vi "Arrange Displays DEMO.vi"() -> ()   [LabVIEW 2016]
uses:
  <vilib>/Utility/miscctls.llb/LVPointTypeDef.ctl
panel:
  in  "stop":bool
  in  "Number of Displays":u8
  in  "Aspect Ratio (Width/Height)":dbl
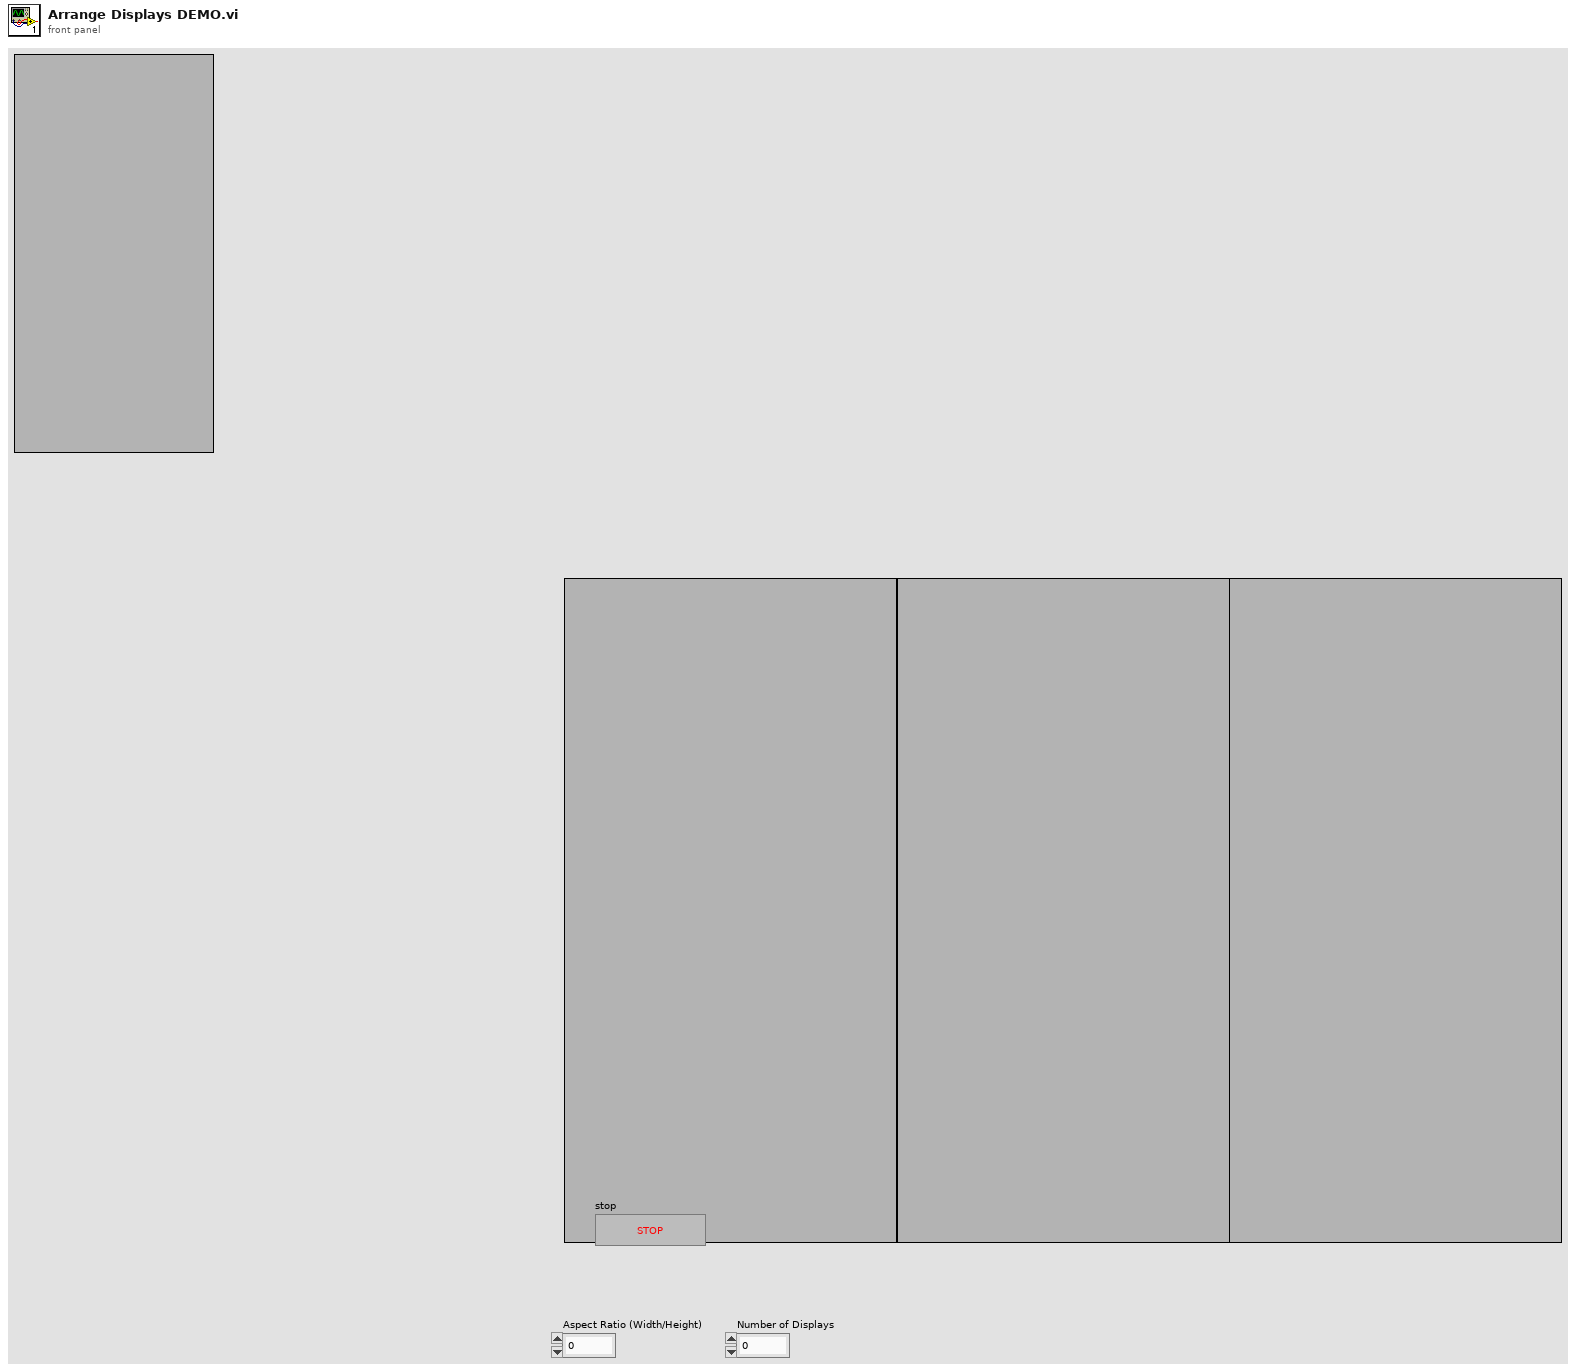
[diagram p1: front panel]
types:
  T1 = enum16{"Always On", "Always Off", "Off While Running"}
  T2 = typedef "LVPointTypeDef.ctl" = cluster{"Horizontal":i16, "Vertical":i16}
  T3 = typedef "LVRectTypeDef.ctl" = cluster{"Left":i16, "Top":i16, "Right":i16, "Bottom":i16}
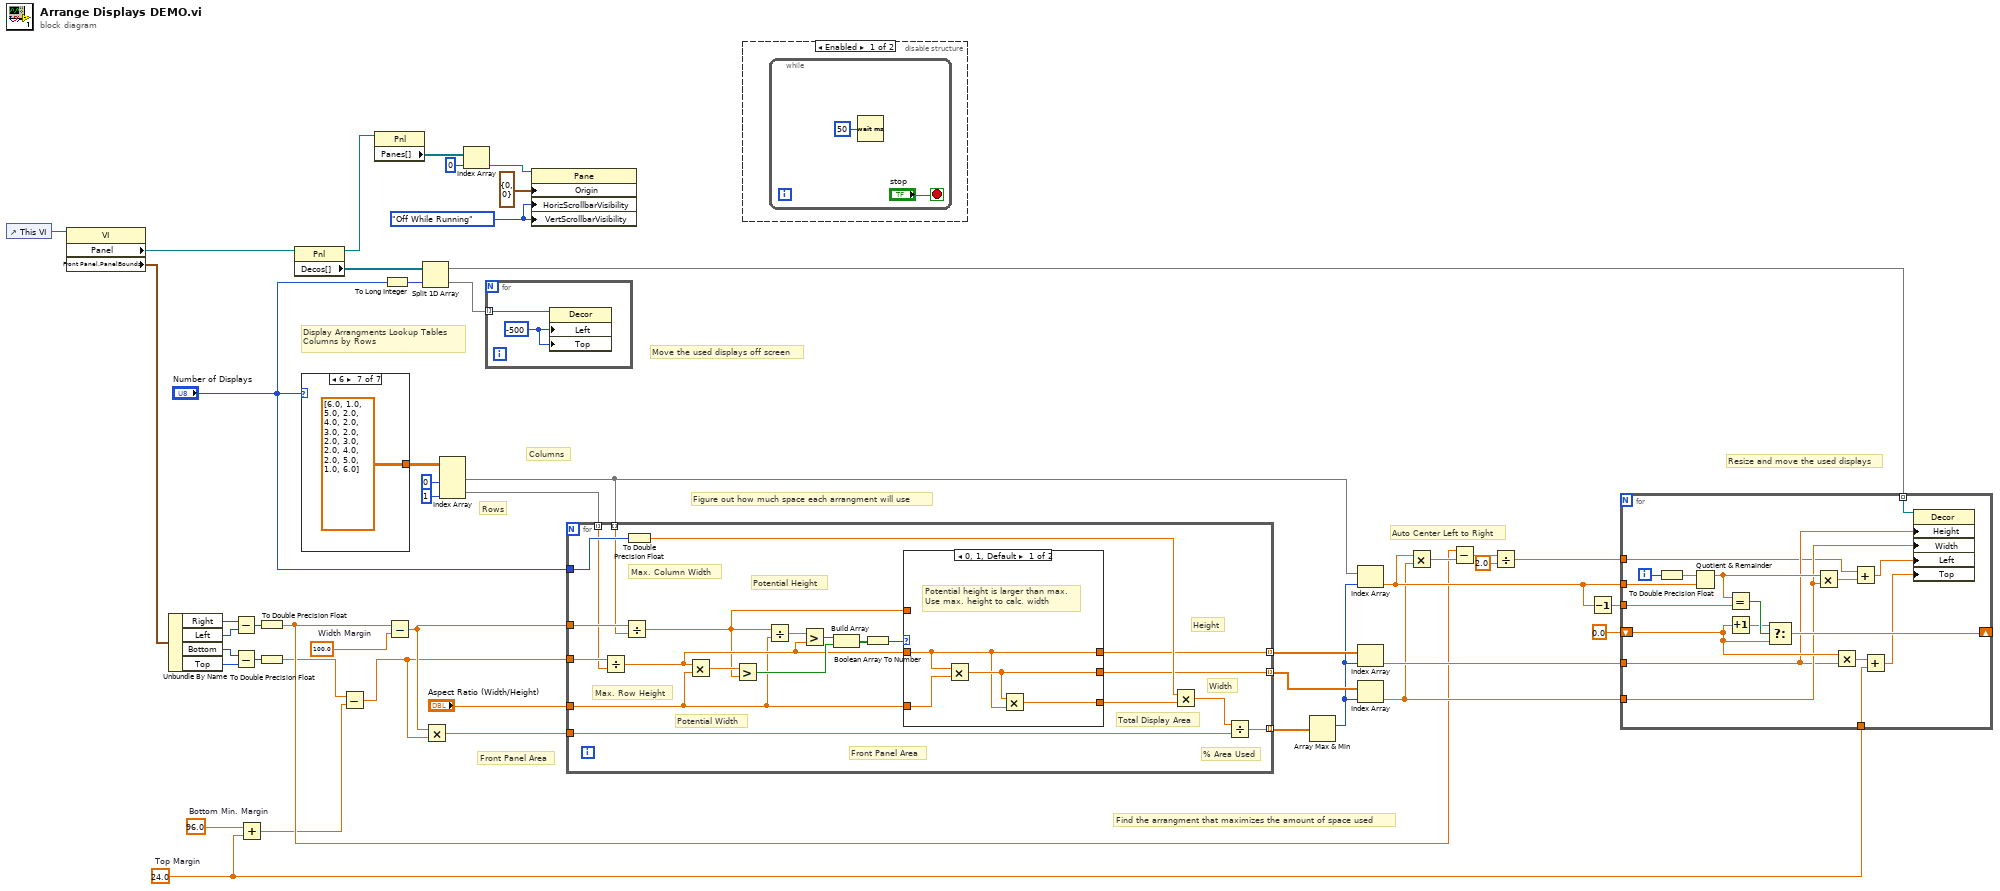
[diagram p0: block diagram]
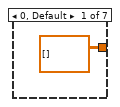
[diagram p3: hidden frame]
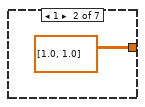
[diagram p4: hidden frame]
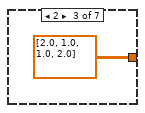
[diagram p5: hidden frame]
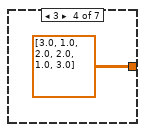
[diagram p6: hidden frame]
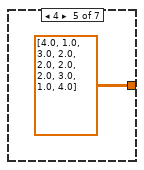
[diagram p7: hidden frame]
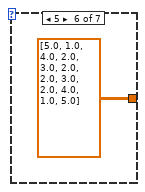
[diagram p8: hidden frame]
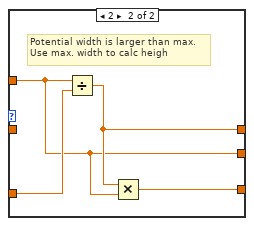
[diagram p9: hidden frame]
diagram:
  w1 = 96.0  # Bottom Min. Margin
  w5 = 24.0  # Top Margin
  w14 = 100.0  # Width Margin
  w42 = T1."Off While Running" ("Vertical Scrollbar Visibility")
  # "Auto Center Left to Right"
  # "Resize and move the used displays"
  # "Find the arrangment that maximizes the amount of space used"
  # "Figure out how much space each arrangment will use"
  # "Move the used displays off screen"
  # "Front Panel Area"
  # "Rows"
  # "Columns"
  # "Display Arrangments Lookup Tables\nColumns by Rows"
  n1 = control-ref of="This VI"() -> (w48:refnum<vi>)
  n2 = property class="VI"(reference=w48) -> ("Panel"=w47:refnum<vi>, "Front Panel.PanelBounds"=w40:T3)  [unwired: 1 in, 2 out]
  n3 = Unbundle By Name(w40) -> ("Right"=w39:i16, "Left"=w38:i16, "Bottom"=w37:i16, "Top"=w36:i16)
  n4 = Subtract(x=w39, y=w38) -> (x-y=w34:i16)
  n5 = Subtract(x=w37, y=w36) -> (x-y=w33:i16)
  n6 = Add(x=w1, y=w5) -> (x+y=w4:dbl)
  n7 = To Double Precision Float(number=w34) -> (double precision float=w6:dbl)
  n8 = To Double Precision Float(number=w33) -> (double precision float=w3:dbl)
  n9 = property class="Pnl"(reference=w47) -> (reference out=w41:refnum<vi>, "Decos[]"=w19:refnum<vi>[])  [unwired: 1 in, 1 out]
  n10 = case shown="6" "Number of Displays" {
    tunnel: [dbl[][] [] dbl[][] [[1.0, 1.0]] dbl[][] [[2.0, 1.0], [1.0, 2.0]] dbl[][] [[3.0, 1.0], [2.0, 2.0], [1.0, 3.0]] dbl[][] [[4.0, 1.0], [3.0, 2.0], [2.0, 2.0], [2.0, 3.0], [1.0, 4.0]] dbl[][] [[5.0, 1.0], [4.0, 2.0], [3.0, 2.0], [2.0, 3.0], [2.0, 4.0], [1.0, 5.0]] dbl[][] [[6.0, 1.0], [5.0, 2.0], [4.0, 2.0], [3.0, 2.0], [2.0, 3.0], [2.0, 4.0], [2.0, 5.0], [1.0, 6.0]]] -> w31
    frame 0, Default {
    }
    frame 1 {
    }
    frame 2 {
    }
    frame 3 {
    }
    frame 4 {
    }
    frame 5 {
    }
    frame 6 {
    }
  }
  n11 = Subtract(x=w3, y=w4) -> (x-y=w2:dbl)
  n12 = property class="Pnl"(reference=w41) -> ("Panes[]"=w46:refnum<vi>[])  [unwired: 1 in, 2 out]
  n13 = To Long Integer(number="Number of Displays") -> (32bit integer=w17:i32)
  n14 = Subtract(x=w6, y=w14) -> (x-y=w13:dbl)
  n15 = Split 1D Array(array=w19, index=w17) -> (first subarray=w18:refnum<vi>[], second subarray=w16:refnum<vi>[])
  n16 = Multiply(x=w13, y=w2) -> (x*y=w32:dbl)
  n17 = Index Array(array=w31, index (col) #1=0 ("disabled index (col)"), index (col) #2=1 ("index (col)")) -> (element #1=w24:dbl[], element #2=w23:dbl[])  [unwired: 2 in]
  n18 = Index Array(array=w46, index=0) -> (element=w44:refnum<vi>)
  n19 = for {
    tunnel: w16 -> [w57] mode=indexing
    w56 = -500 ("Position:Left")
    n20 = property class="Decor"(reference=w57, "Left"=w56, "Top"=w56) -> ()  [unwired: 1 in, 2 out]
  }
  n21 = property class="Pane"(reference=w44, "Origin"=T2 {"Horizontal"=0, "Vertical"=0}, "HorizScrollbarVisibility"=w42, "VertScrollbarVisibility"=w42) -> ()  [unwired: 1 in, 2 out]
  n22 = for {
    tunnel: "Aspect Ratio (Width/Height)" -> [w69]
    tunnel: w13 -> [w78]
    tunnel: w2 -> [w77]
    tunnel: w32 -> [w63]
    tunnel: [w66] -> w27 mode=indexing
    tunnel: [w65] -> w26 mode=indexing
    tunnel: [w62] -> w28 mode=indexing
    tunnel: w24 -> [w59] mode=indexing
    tunnel: w23 -> [w58] mode=indexing
    tunnel: "Number of Displays" -> [w60]
    # "% Area Used"
    # "Front Panel Area"
    # "Total Display Area"
    # "Width"
    # "Height"
    # "Potential Height"
    # "Potential Width"
    # "Max. Row Height"
    # "Max. Column Width"
    n23 = Divide(x=w77, y=w58) -> (x/y=w71:dbl)
    n24 = Divide(x=w78, y=w59) -> (x/y=w70:dbl)
    n25 = To Double Precision Float(number=w60) -> (double precision float=w67:dbl)
    n26 = Multiply(x=w71, y=w69) -> (x*y=w76:dbl)
    n27 = Greater?(x=w76, y=w70) -> (0:w73:bool)
    n28 = Divide(x=w70, y=w69) -> (x/y=w75:dbl)
    n29 = Greater?(x=w75, y=w71) -> (0:w74:bool)
    n30 = Build Array(w74, w73) -> (w72:bool[])
    n31 = Boolean Array To Number(Boolean array=w72) -> (number=w61:u32)
    n32 = case shown="0, 1, Default" w61 {
      tunnel: w71 -> [w80 _]
      tunnel: w70 -> [_ w84]
      tunnel: w69 -> [w82 w86]
      tunnel: [w80 w85] -> w66
      tunnel: [w81 w84] -> w65
      tunnel: [w79 w83] -> w68
      frame 0, 1, Default {
        # "Potential height is larger than max.\nUse max. height to calc. width"
        n33 = Multiply(x=w80, y=w82) -> (x*y=w81:dbl)
        n34 = Multiply(x=w81, y=w80) -> (x*y=w79:dbl)
      }
      frame 2 {
        # "Potential width is larger than max.\nUse max. width to calc heigh"
        n35 = Divide(x=w84, y=w86) -> (x/y=w85:dbl)
        n36 = Multiply(x=w85, y=w84) -> (x*y=w83:dbl)
      }
    }
    n37 = Multiply(x=w67, y=w68) -> (x*y=w64:dbl)
    n38 = Divide(x=w64, y=w63) -> (x/y=w62:dbl)
  }
  n39 = disable-structure shown="Enabled" {
    frame Enabled {
      n40 = while {
        stop <- "stop" stop-if-true
        n41 = Wait (ms)(milliseconds to wait=u32 50) -> ()  [unwired: 1 out]
      }
    }
    frame Disabled {
    }
  }
  n42 = Array Max & Min(array=w28) -> (max index (indices)=w22:i32)  [unwired: 3 out]
  n43 = Index Array(array=w24, index=w22) -> (element=w12:dbl)
  n44 = Index Array(array=w27, index=w22) -> (element=w25:dbl)
  n45 = Index Array(array=w26, index=w22) -> (element=w11:dbl)
  n46 = Multiply(x=w12, y=w11) -> (x*y=w10:dbl)
  n47 = Subtract(x=w6, y=w10) -> (x-y=w9:dbl)
  n48 = Divide(x=w9, y=2.0) -> (x/y=w7:dbl)
  n49 = Decrement(x=w12) -> (x-1=w21:dbl)
  n50 = for {
    tunnel: w25 -> [w95]
    tunnel: w11 -> [w96]
    tunnel: w12 -> [w106]
    tunnel: w18 -> [w97] mode=indexing
    tunnel: w21 -> [w103]
    shift-right: [w100] -> _
    shift-left: 0.0 -> [w99]
    tunnel: w7 -> [w93]
    tunnel: w5 -> [w90]
    i -> [w104]
    n51 = To Double Precision Float(number=w104) -> (double precision float=w105:dbl)
    n52 = Quotient & Remainder(x=w105, y=w106) -> (x-y*floor(x/y)=w98:dbl)  [unwired: 1 out]
    n53 = Equal?(x=w98, y=w103) -> (x = y?=w102:bool)
    n54 = Increment(x=w99) -> (x+1=w101:dbl)
    n55 = Select(t=w101, s=w102, f=w99) -> (s? t:f=w100:dbl)
    n56 = Multiply(x=w98, y=w96) -> (x*y=w94:dbl)
    n57 = Multiply(x=w99, y=w95) -> (x*y=w91:dbl)
    n58 = Add(x=w93, y=w94) -> (x+y=w92:dbl)
    n59 = Add(x=w91, y=w90) -> (x+y=w89:dbl)
    n60 = property class="Decor"(reference=w97, "Height"=w95, "Width"=w96, "Left"=w92, "Top"=w89) -> ()  [unwired: 1 in, 2 out]
  }
